vi "GEA2 Script_Log Header.vi"(0 "Filename":string, 7 "# of Test Cases":i32, 11 "Version":string) -> (8 "Header":string)   [LabVIEW 2014]
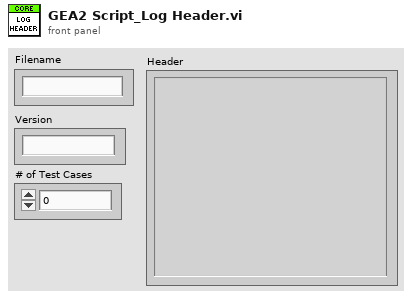
[diagram p1: front panel]
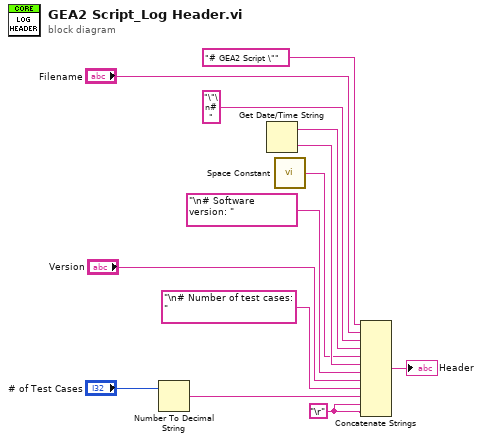
[diagram p0: block diagram]
diagram:
  w1 = "\r"
  n1 = Number To Decimal String(number="# of Test Cases") -> (decimal integer string=w2:string)  [unwired: 1 in]
  n2 = Get Date/Time String() -> (date string=w13:string, time string=w12:string)  [unwired: 3 in]
  n3 = call <vilib>:"Space Constant.vi"() -> ("String"=w11:string)
  n4 = Concatenate Strings("# GEA2 Script \"", "Filename", "\"\n# " ("string"), w13, w11, w12, "\n# Software version: " ("string"), "Version", "\n# Number of test cases: " ("string"), w2, w1, w1) -> (→"Header":string)
